vi "Initialize NI-DAQ digitizer.vi"(8 "error in (no error)":errorcluster, 11 "Parameters":T1={"physical channels"="Dev1/ai0:7", "input terminal configuration"=10106, "Range"=10.0, "Sample rate"=1000000.0, "samples per channel"=220000, "Trigger source"="/Dev1/PFI0", "pretrigger samples per channel"=20000, "task"="", "Sample mode"=10178, "Retriggerable"=FALSE} {"Sample mode" items=["Finite Samples"=10178, "Continuous Samples"=10123, "Hardware Timed Single Point"=12522]; "Sample rate" format="%.2p"; "input terminal configuration" items=["default"=-1, "RSE"=10083, "NRSE"=10078, "Differential"=10106, "Pseudodifferential"=12529]}) -> (0 "error out":errorcluster, 3 "Parameters out":T1={"physical channels"="Dev1/ai0:7", "input terminal configuration"=10106, "Range"=10.0, "Sample rate"=1000000.0, "samples per channel"=220000, "Trigger source"="/Dev1/PFI0", "pretrigger samples per channel"=20000, "task"="", "Sample mode"=10178, "Retriggerable"=FALSE} {"Sample mode" items=["Finite Samples"=10178, "Continuous Samples"=10123, "Hardware Timed Single Point"=12522]; "Sample rate" format="%.2p"; "input terminal configuration" items=["default"=-1, "RSE"=10083, "NRSE"=10078, "Differential"=10106, "Pseudodifferential"=12529]})   [LabVIEW 2015]
uses:
  NI-DAQ digitizer parameters.ctl
  <vilib>/DAQmx/create/channels.llb/DAQmx Create Channel (AI-Voltage-Basic).vi
  <vilib>/DAQmx/configure/timing.llb/DAQmx Timing (Sample Clock).vi
  <vilib>/DAQmx/configure/trigger.llb/DAQmx Reference Trigger (Digital Edge).vi
  <resource>/objmgr/daqmx.rc
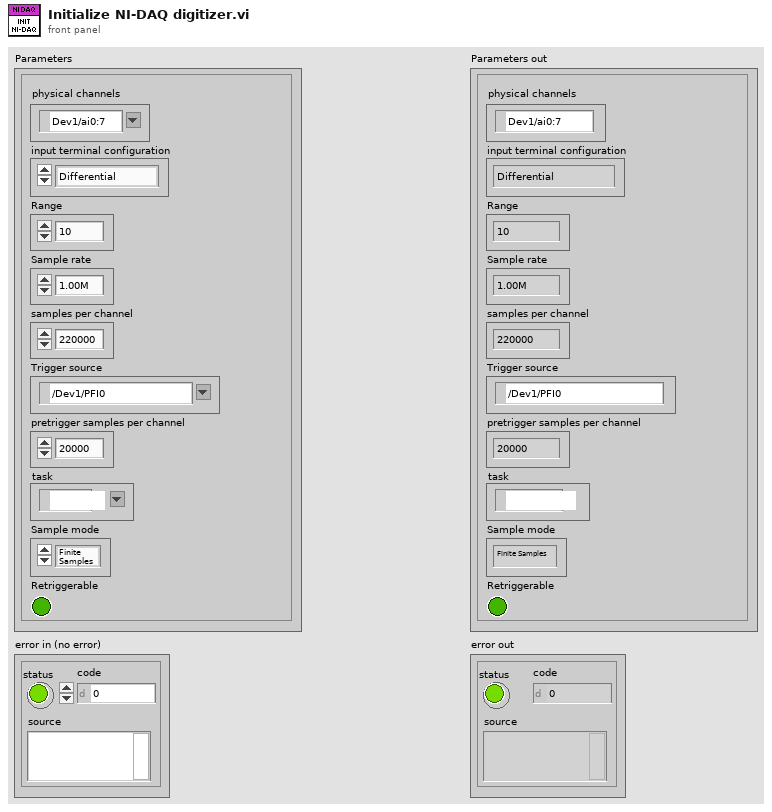
[diagram p1: front panel]
types:
  T1 = typedef "NI-DAQ digitizer parameters.ctl" = cluster{"physical channels":tag, "input terminal configuration":i32, "Range":dbl, "Sample rate":dbl, "samples per channel":i32, "Trigger source":tag, "pretrigger samples per channel":u32, "task":refnum<k21>, "Sample mode":i32, "Retriggerable":bool}
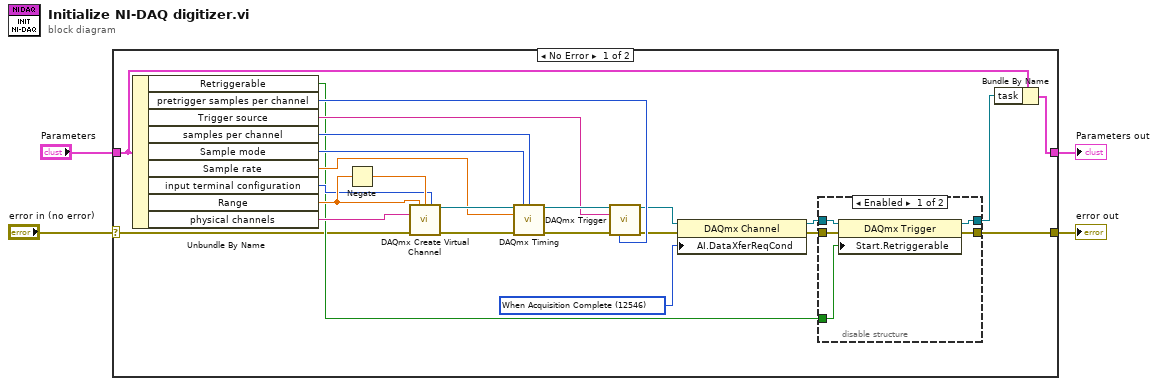
[diagram p0: block diagram]
diagram:
  n1 = case shown="No Error" "error in (no error)" {
    selector: "error in (no error)" -> [w5 w37]
    tunnel: [w23 w37] -> w1
    tunnel: [w13 w36] -> w2
    tunnel: "Parameters" -> [w6 w36]
    frame No Error {
      w11 = 12546 items=["Onboard Memory More than Half Full"=10237, "Onboard Memory Not Empty"=10241, "Onboard Memory Custom Threshold"=12577, "When Acquisition Complete"=12546] ("AI.DataXferReqCond")
      n2 = Unbundle By Name(w6) -> ("Retriggerable"=w14:bool, "pretrigger samples per channel"=w15:u32, "Trigger source"=w16:tag, "samples per channel"=w17:i32, "Sample mode"=w18:i32, "Sample rate"=w19:dbl, "input terminal configuration"=w20:i32, "Range"=w21:dbl, "physical channels"=w22:tag)
      n3 = Negate(x=w21) -> (-x=w28:dbl)
      n4 = call-poly <vilib>:"DAQmx Create Virtual Channel.vi"("maximum value"=w21, "minimum value"=w28, "input terminal configuration"=w20, "physical channels"=w22, "error in"=w5) -> ("task out"=w27:refnum<k21>, "error out"=w26:errorcluster)  [unwired: 4 in, 5 out]
      n5 = call-poly <vilib>:"DAQmx Timing.vi"("task/channels in"=w27, "sample mode"=w18, "samples per channel"=w17, "rate"=w19, "error in"=w26) -> ("task out"=w25:refnum<k21>, "error out"=w24:errorcluster)  [unwired: 9 in]
      n6 = call-poly <vilib>:"DAQmx Trigger.vi"("task/channels in"=w25, "source"=w16, "error in"=w24, "pretrigger samples per channel"=w15) -> ("task out"=w10:refnum<k21>, "error out"=w7:errorcluster)  [unwired: 1 in, 9 out]
      n7 = property class="DAQmx Channel"(reference=w10, error in=w7, "AI.DataXferReqCond"=w11) -> (reference out=w9:refnum<k21>, error out=w8:errorcluster)
      n8 = disable-structure shown="Enabled" {
        disable-tunnel: w8 -> [w33 w35]
        disable-tunnel: w9 -> [w32 w34]
        disable-tunnel: [w31 w35] -> w23
        disable-tunnel: w14 -> [w30 _]
        disable-tunnel: [w29 w34] -> w12
        frame Enabled {
          n9 = property class="DAQmx Trigger"(reference=w32, error in=w33, "Start.Retriggerable"=w30) -> (reference out=w29:refnum<k21>, error out=w31:errorcluster)
        }
        frame Disabled {
        }
      }
      n10 = Bundle By Name(cluster=w6, "task"=w12) -> (w13:T1)
    }
    frame Error {
    }
  }
  "error out" <- w1
  "Parameters out" <- w2
